vi "Edge.vi"(8 "Index2":i32, 9 "Index1":i32, 10 "Slope":dbl, 11 "DocIn":refnum<k20>) -> (2 "Edge":refnum<k20>, 3 "DocOut":refnum<k20>)   [LabVIEW 2014]
uses:
  <resource>/objmgr/DOMUserDefRef.rc
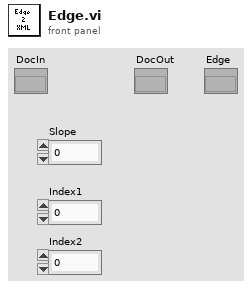
[diagram p1: front panel]
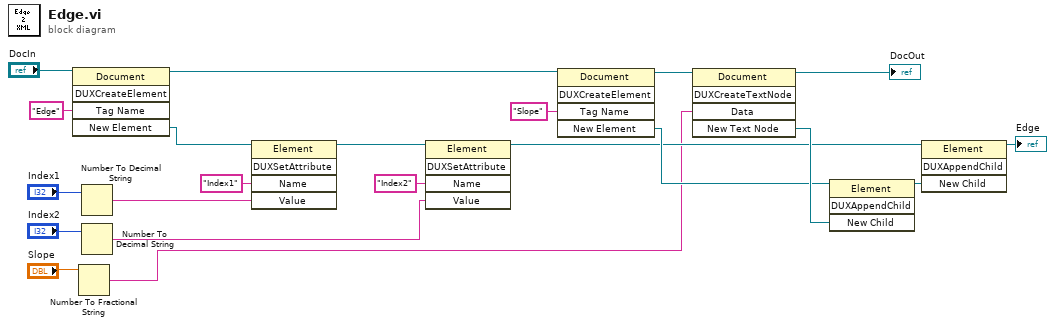
[diagram p0: block diagram]
diagram:
  n1 = invoke class="Document" method="DUXCreateElement"(reference="DocIn", "Tag Name"="Edge") -> (reference out=w15:refnum<k20>, "New Element"=w16:refnum<k20>)  [unwired: 3 in, 3 out]
  n2 = Number To Fractional String(number="Slope") -> (F-format string=w4:string)  [unwired: 3 in]
  n3 = Number To Decimal String(number="Index1") -> (decimal integer string=w13:string)  [unwired: 1 in]
  n4 = Number To Decimal String(number="Index2") -> (decimal integer string=w6:string)  [unwired: 1 in]
  n5 = invoke class="Element" method="DUXSetAttribute"(reference=w16, "Name"="Index1", "Value"=w13) -> (reference out=w7:refnum<k20>)  [unwired: 2 in, 4 out]
  n6 = invoke class="Element" method="DUXSetAttribute"(reference=w7, "Name"="Index2", "Value"=w6) -> (reference out=w5:refnum<k20>)  [unwired: 2 in, 4 out]
  n7 = invoke class="Document" method="DUXCreateElement"(reference=w15, "Tag Name"="Slope") -> (reference out=w19:refnum<k20>, "New Element"=w17:refnum<k20>)  [unwired: 3 in, 3 out]
  n8 = invoke class="Document" method="DUXCreateTextNode"(reference=w19, "Data"=w4) -> (reference out=→"DocOut":refnum<k20>, "New Text Node"=w18:refnum<k20>)  [unwired: 3 in, 3 out]
  n9 = invoke class="Element" method="DUXAppendChild"(reference=w17, "New Child"=w18) -> (reference out=w11:refnum<k20>)  [unwired: 2 in, 3 out]
  n10 = invoke class="Element" method="DUXAppendChild"(reference=w5, "New Child"=w11) -> (reference out=→"Edge":refnum<k20>)  [unwired: 2 in, 3 out]
